vi "HMS_to Seconds.vi"(11 "H:M:S":string) -> (2 "double precision float":dbl, 3 "Second":i32)   [LabVIEW 2021]
doc: "24小时格式的时分秒转换为对应的秒。\n# 2020-7-7 15:26:14"
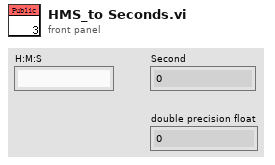
[diagram p1: front panel]
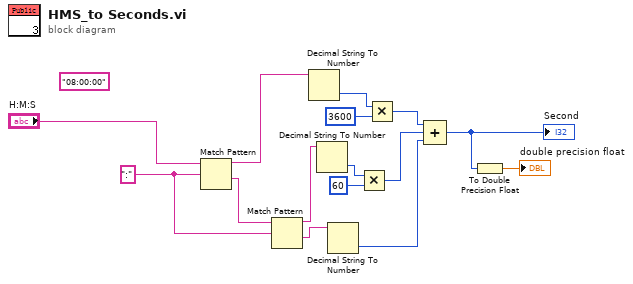
[diagram p0: block diagram]
diagram:
  (unwired) "08:00:00" ("time format string (%c)")
  w5 = ":" ("regular expression")
  n1 = Match Pattern(string="H:M:S", regular expression=w5) -> (before substring=w8:string, after substring=w4:string)  [unwired: 1 in, 2 out]
  n2 = Match Pattern(string=w4, regular expression=w5) -> (before substring=w11:string, after substring=w12:string)  [unwired: 1 in, 2 out]
  n3 = Decimal String To Number(string=w8) -> (number=w7:i32)  [unwired: 2 in, 1 out]
  n4 = Decimal String To Number(string=w11) -> (number=w9:i32)  [unwired: 2 in, 1 out]
  n5 = Decimal String To Number(string=w12) -> (number=w15:i32)  [unwired: 2 in, 1 out]
  n6 = Multiply(x=w9, y=60) -> (x*y=w14:i32)
  n7 = Multiply(x=w7, y=3600) -> (x*y=w13:i32)
  n8 = Compound Arithmetic op=ADD(w13, w14, w15) -> (w2:i32)
  "Second" <- w2
  n9 = To Double Precision Float(number=w2) -> (double precision float=→"double precision float":dbl)
